vi "DIO Read.vi"(2 "Channels":i32[](array[numeric]), 3 "device":i16=1) -> (0 "Error":bool, 1 "Data":bool[](array[boolean]))   [LabVIEW 2009]
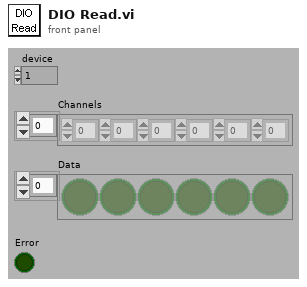
[diagram p1: front panel]
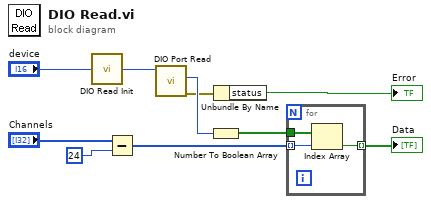
[diagram p0: block diagram]
diagram:
  n1 = call "DIO Read Init.vi"("device"="device") -> ("task ID out"=w2:u32)
  n2 = Subtract(x="Channels", y=i16 24 ("port width")) -> (x-y=w4:i32[])
  n3 = call <vilib>:"DIO Port Read.vi"("task ID"=w2) -> ("error out"=w8:errorcluster, "pattern"=w10:u32)  [unwired: 8 in, 1 out]
  n4 = Number To Boolean Array(number=w10) -> (Boolean array=w3:bool[])
  n5 = Unbundle By Name(w8) -> ("status"=→"Error":bool)
  n6 = for {
    tunnel: w3 -> [w13]
    tunnel: w4 -> [w12] mode=indexing
    tunnel: [w11] -> w9 mode=indexing
    n7 = Index Array(array=w13, index=w12) -> (element=w11:bool)
  }
  "Data" <- w9
